vi "ServerGlobals.vi"() -> ()   [LabVIEW 2017, in "Server.lvlib"]
uses:
  Server.lvlib
panel:
  out "Stop?":bool
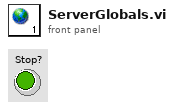
[diagram p1: front panel]
diagram:
